vi "Channel Monitor (simulated data).vi"() -> ()   [LabVIEW 2011]
doc: "This example shows how the Channel Monitor XControl can be used to view signal levels. The levels shown in the meter are RMS levels\nwhich is why the Sine, Square, and Triangle show different levels for the same amplitude signal.\n\nSome things to try:\n-To view the actual time domain signal, you can click on an associated button to launch a display.\n-Expand the XControl vertical to add more visible rows.\n-In edit time, right-click the XControl and select \"Change Level Color\" to change the color of the bars."
uses:
  user.lib/Channel Monitor/Channel Monitor.xctl
  <vilib>/measure/NI_MABase.lvlib
panel:
  in  "Amplitude":dbl(knob)=1.5 scale=0.0..10.0
  in  "Frequency":dbl(knob)=25.0 scale=0.0..100.0
  in  "stop":bool
  out "Channel Monitor":waveform(dbl)[](xcontrol)
  # "This example shows how the Channel Monitor XControl can be used to view signal levels. \n\nSome things to try:\n-To view the actual time domain signal, you can click on an associated button to launch a display.\n-Expand the XControl vertical to add more visible rows.\n-In edit time, right-click the XControl and select \"Change Level Color\" to change the color of the bars."
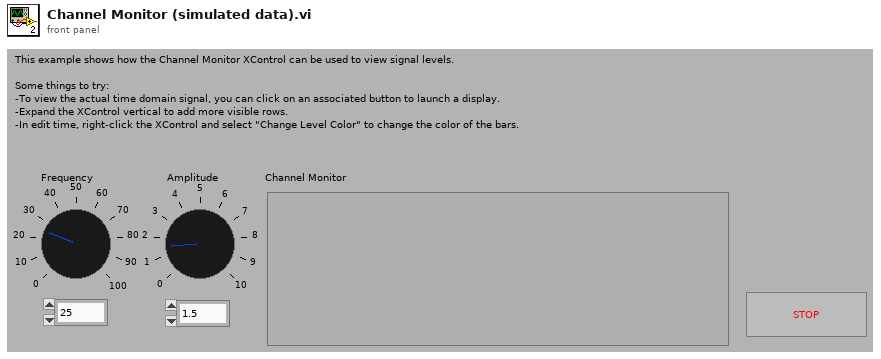
[diagram p1: front panel]
types:
  T1 = enum16{"Sine Wave", "Triangle Wave", "Square Wave", "Sawtooth Wave"}[]
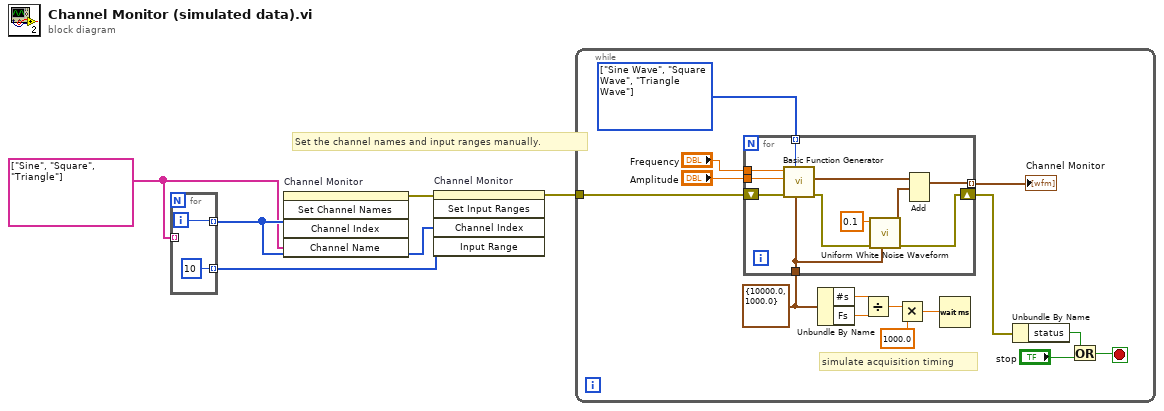
[diagram p0: block diagram]
diagram:
  w2 = string[] ["Sine", "Square", "Triangle"] ("Channel Name")
  # "Set the channel names and input ranges manually."
  n1 = for {
    tunnel: [w7] -> w3 mode=indexing
    tunnel: w2 -> [_] mode=indexing
    tunnel: [10] -> w1 mode=indexing
    i -> [w7]
  }
  n2 = invoke on="Channel Monitor" class="Channel Monitor (strict)" method="Set Channel Names"("Channel Index"=w3, "Channel Name"=w2) -> (error out=w5:errorcluster)  [unwired: 3 in, 4 out]
  n3 = invoke on="Channel Monitor" class="Channel Monitor (strict)" method="Set Input Ranges"(error in=w5, "Channel Index"=w3, "Input Range"=w1) -> (error out=w4:errorcluster)  [unwired: 2 in, 4 out]
  n4 = while {
    tunnel: w4 -> [w21]
    stop <- w15 stop-if-true
    w22 = T1 [enum."Sine Wave", enum."Square Wave", enum."Triangle Wave"] items=["Sine Wave", "Triangle Wave", "Square Wave", "Sawtooth Wave"]
    w18 = cluster{"Fs":dbl, "#s":dbl} {"Fs"=10000.0, "#s"=1000.0} ("sampling info")
    # "simulate acquisition timing"
    n5 = for {
      tunnel: w18 -> [w33]
      tunnel: w22 -> [w29] mode=indexing
      tunnel: [w25] -> w8 mode=indexing
      shift-right: [w26] -> w12
      shift-left: w21 -> [w28]
      tunnel: "Frequency" -> [w24]
      tunnel: "Amplitude" -> [w23]
      n6 = call <vilib>:"Basic Function Generator.vi"("sampling info"=w33, "signal type"=w29, "error in (no error)"=w28, "amplitude"=w23, "frequency"=w24) -> ("error out"=w27:errorcluster, "signal out"=w32:waveform(dbl))  [unwired: 4 in, 1 out]
      n7 = call <vilib>:"Uniform White Noise Waveform.vi"("sampling info"=w33, "error in (no error)"=w27, "amplitude"=0.1) -> ("error out"=w26:errorcluster, "signal out"=w31:waveform(dbl))  [unwired: 7 in]
      n8 = Add(1:w31, 2:w32) -> (0:w25:waveform(dbl))  [unwired: 1 in, 1 out]
    }
    "Channel Monitor" <- w8
    n9 = Unbundle By Name(w18) -> ("#s"=w16:dbl, "Fs"=w17:dbl)
    n10 = Divide(x=w16, y=w17) -> (x/y=w11:dbl)
    n11 = Multiply(x=w11, y=1000.0) -> (x*y=w10:dbl)
    n12 = Wait (ms)(milliseconds to wait=w10) -> ()  [unwired: 1 out]
    n13 = Unbundle By Name(w12) -> ("status"=w13:bool)
    n14 = Or(x=w13, y="stop") -> (x .or. y?=w15:bool)
  }
